vi "Lecroy_clear_buffer.vi"(2 "Inst_parameters":T1={"Kind"=enum."LeCroy", "Strings"=["LeCroy", "192.168.137.1", "F2", "V", "9", "1.0"], "uint64s"=[1, 12, 4, 0, 1, 2, 2], "Doubles"=[], "DAQmx take out list"=[]}) -> ()   [LabVIEW 2013]
uses:
  FPGA-clean_works_1.19f  - Matlab disabled/fpga-clean/host-subVIs/LeCroy Wave Series/LeCroy Wave Series.lvlib
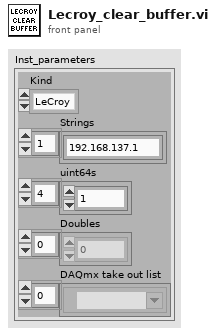
[diagram p1: front panel]
types:
  T1 = cluster{"Kind":enum16{"ADC", "K2000", "34401A", "LeCroy"}, "Strings":string[], "uint64s":u64[], "Doubles":dbl[], "DAQmx take out list":refnum<k21>[]}
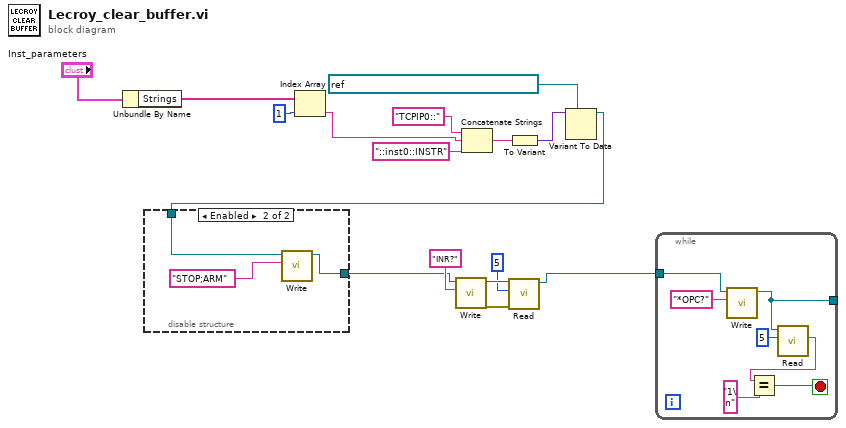
[diagram p0: block diagram]
diagram:
  n1 = Unbundle By Name("Inst_parameters") -> ("Strings"=w15:string[])
  n2 = Index Array(array=w15, index=1) -> (element=w8:string)
  n3 = Concatenate Strings("TCPIP0::" ("string"), w8, "::inst0::INSTR" ("string")) -> (w13:string)
  n4 = To Variant(anything=w13) -> (Variant=w10:variant)
  n5 = Variant To Data(type=refnum<visa-resource-name> "TCPIP0::192.168.137.3::inst0::INSTR" ("VISA resource name"), Variant=w10) -> (data=w7:refnum<visa-resource-name>)  [unwired: 1 in, 1 out]
  n6 = disable-structure shown="Enabled" {
    disable-tunnel: w7 -> [w17 w19]
    disable-tunnel: [w17 w18] -> w2
    frame Disabled {
    }
    frame Enabled {
      n7 = call "Write.vi"("Write Buffer"="STOP;ARM" ("write buffer"), "VISA resource name"=w19) -> ("VISA resource name out"=w18:refnum<visa-resource-name>)  [unwired: 1 in, 8 out]
    }
  }
  n8 = call "Write.vi"("Write Buffer"="INR?" ("write buffer"), "VISA resource name"=w2) -> ("error out"=w5:errorcluster, "VISA resource name out"=w6:refnum<visa-resource-name>)  [unwired: 1 in, 7 out]
  n9 = call "Read.vi"("error in (no error)"=w5, "Byte Count"=u32 5 ("byte count"), "VISA resource name"=w6) -> ("VISA resource name out"=w1:refnum<visa-resource-name>)  [unwired: 8 out]
  n10 = while {
    tunnel: w1 -> [w26]
    tunnel: [w21] -> _
    stop <- w23 stop-if-true
    n11 = call "Write.vi"("Write Buffer"="*OPC?", "VISA resource name"=w26) -> ("VISA resource name out"=w21:refnum<visa-resource-name>)  [unwired: 1 in, 8 out]
    n12 = call "Read.vi"("Byte Count"=u32 5, "VISA resource name"=w21) -> ("Read Buffer"=w24:string)  [unwired: 1 in, 8 out]
    n13 = Equal?(x=w24, y="1\n") -> (x = y?=w23:bool)
  }
